vi "Vision_sRGBToCIE(XYZ).vi"(8 "error in":errorcluster, 9 "Blue":u8, 10 "Green":u8, 11 "Red":u8) -> (0 "error out":errorcluster, 1 "Z":dbl format="%.6f", 2 "Y":dbl format="%.6f", 3 "X":dbl format="%.6f", 4 "y":dbl format="%.6f", 5 "x":dbl format="%.6f", 6 "Y":dbl format="%.6f")   [LabVIEW 2013]
doc: "Converts an RGB color value into another format (HSL, HSV, HSI, CIE L*a*b*, or CIE XYZ)."
uses:
  <vilib>/Analysis/Matrix/Datatypes/RealMatrix.ctl
  <vilib>/Analysis/baseanly.llb/Real A x B.vi
  <vilib>/Analysis/NI_AALBase.lvlib
  <vilib>/Analysis/Matrix/NI_Matrix.lvlib
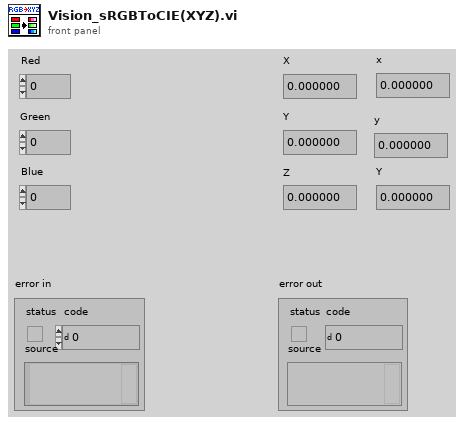
[diagram p1: front panel]
types:
  T1 = typedef "NI_Matrix.lvlib/RealMatrix.ctl" = dbl[][]
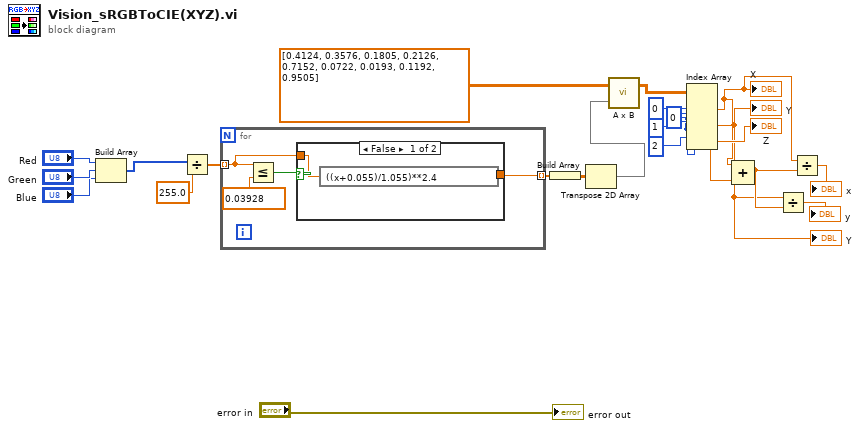
[diagram p0: block diagram]
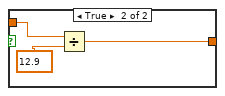
[diagram p2: hidden frame]
diagram:
  w7 = 0
  n1 = Build Array("Red", "Green", "Blue") -> (w12:u8[])
  n2 = Divide(x=w12, y=255.0) -> (x/y=w19:dbl[])
  n3 = for {
    tunnel: w19 -> [w24] mode=indexing
    tunnel: [w23] -> w18 mode=indexing
    n4 = Less Or Equal?(x=w24, y=0.03928) -> (x <= y?=w25:bool)
    n5 = case shown="False" w25 {
      tunnel: w24 -> [w28 w30]
      tunnel: [w27 w29] -> w23
      frame False {
        n6 = expression code="((x+0.055)/1.055)**2.4"(w28) -> (w27:dbl)
      }
      frame True {
        n7 = Divide(x=w30, y=12.9) -> (x/y=w29:dbl)
      }
    }
  }
  n8 = Build Array(w18) -> (w17:dbl[][])
  n9 = Transpose 2D Array(2D array=w17) -> (transposed array=w16:dbl[][])
  n10 = call-poly <vilib>:"A x B.vi"("B"=w16, "A"=T1 [[0.4124, 0.3576, 0.1805], [0.2126, 0.7152, 0.0722], [0.0193, 0.1192, 0.9505]]) -> ("A x B"=w11:T1)  [unwired: 1 out]
  n11 = Index Array(array=w11, index (row) #1=0, index (col) #1=w7, index (row) #2=1, index (col) #2=w7, index (row) #3=2, index (col) #3=w7) -> (element #1=w5:dbl, element #2=w1:dbl, element #3=w6:dbl)
  "Z" <- w6
  "Y" <- w1
  "X" <- w5
  "Y" <- w1
  n12 = Compound Arithmetic op=ADD(w5, w1, w6) -> (w2:dbl)
  n13 = Divide(x=w1, y=w2) -> (x/y=→"y":dbl)
  n14 = Divide(x=w5, y=w2) -> (x/y=→"x":dbl)
  "error out" <- "error in"
